vi "Configure Multi Eval Meas List Segment DMRS Type B.vi"(1 "Segment (1)":T3=1, 4 "Max Length (1)":i32=1, 5 "Additional Position (0)":i32, 6 "Config Type (1)":i32=1, 7 "Bandwidth Part (BWP0)":T1 items=["BWP0"], 8 "error in (no error)":errorcluster, 9 "Carrier Component (1)":T2=1, 10 "Instance (1)":T4=1, 11 "VISA resource name":refnum<visa-resource-name>) -> (0 "error out":errorcluster, 3 "VISA resource name out":refnum<visa-resource-name>)   [LabVIEW 2020, in "Rohde&Schwarz CMXP NR FR2 Measurement.lvlib"]
doc: "Configures the DM-RS for mapping type B. The settings apply to the <BWP> on carrier <cc> in segment <no>.\n\nAttribute:\nRSCMXPNRFR2M_ATTR_MULTI_EVAL_MEASUREMENT_LIST_SEGMENT_DMRS_TYPE_B\n\nRemote-control command:\nCONFigure:NRMMw:MEAS<i>:LIST:SEGMent<no>[:CC<cc>]:BWPart:PUSCh:DMTB"
uses:
  <instrlib>/Rohde&Schwarz CMXP NR FR2 Measurement/Rohde&Schwarz CMXP NR FR2 Measurement.lvlib
  <instrlib>/Rohde&Schwarz CMXP NR FR2 Measurement/Private/_Instance.ctl
  <instrlib>/Rohde&Schwarz CMXP NR FR2 Measurement/Private/_Segment.ctl
  <instrlib>/Rohde&Schwarz CMXP NR FR2 Measurement/Private/_Carrier Component.ctl
  <instrlib>/Rohde&Schwarz CMXP NR FR2 Measurement/Private/_Bandwidth Part.ctl
  <instrlib>/Rohde&Schwarz CMXP NR FR2 Measurement/Private/rsidr_core.llb/rsidr_core.lvlib
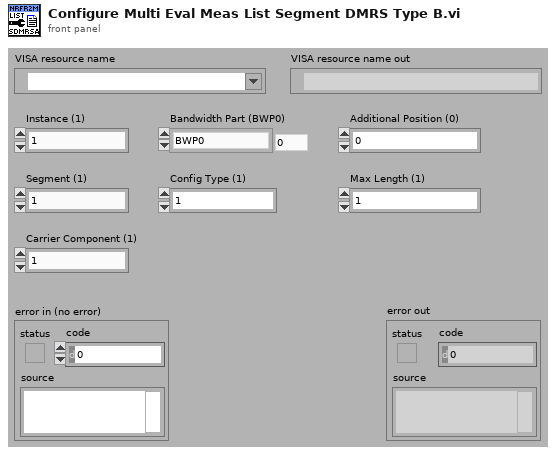
[diagram p1: front panel]
types:
  T1 = typedef "Rohde&Schwarz CMXP NR FR2 Measurement.lvlib/_Bandwidth Part.ctl" = i32
  T2 = typedef "Rohde&Schwarz CMXP NR FR2 Measurement.lvlib/_Carrier Component.ctl" = i32
  T3 = typedef "Rohde&Schwarz CMXP NR FR2 Measurement.lvlib/_Segment.ctl" = i32
  T4 = typedef "Rohde&Schwarz CMXP NR FR2 Measurement.lvlib/_Instance.ctl" = i32
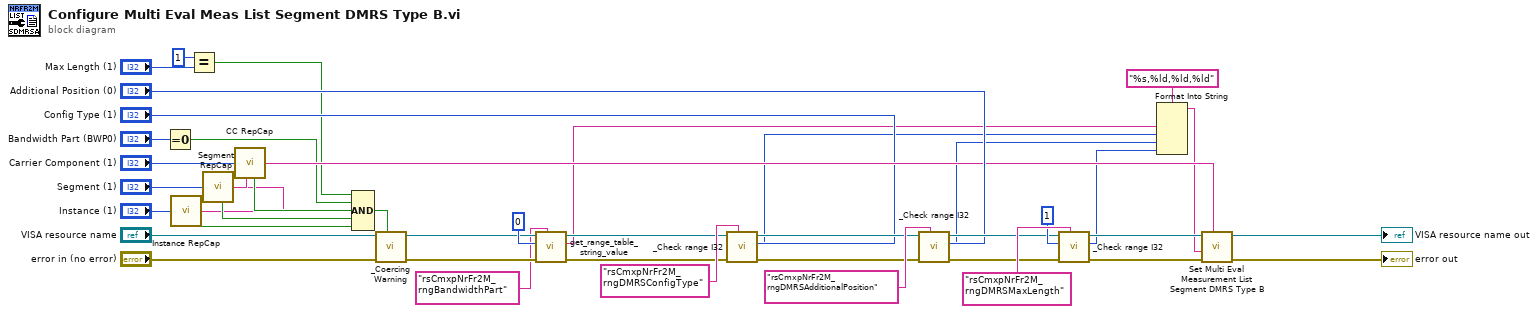
[diagram p0: block diagram]
diagram:
  n1 = Equal To 0?(x="Bandwidth Part (BWP0)") -> (x = 0?=w5:bool)
  n2 = call <instrlib>:"Instance RepCap.vi"("Instance In"="Instance (1)") -> ("In Range?"=w26:bool, "RepCap Identifier Out"=w2:string)  [unwired: 1 in]
  n3 = Equal?(x=1, y="Max Length (1)") -> (x = y?=w4:bool)
  n4 = call <instrlib>:"Segment RepCap.vi"("Segment In"="Segment (1)", "RepCap String In (\"\")"=w2) -> ("In Range?"=w25:bool, "RepCap Identifier Out"=w24:string)
  n5 = call <instrlib>:"CC RepCap.vi"("CC In"="Carrier Component (1)", "RepCap String In (\"\")"=w24) -> ("In Range?"=w23:bool, "RepCap Identifier Out"=w11:string)
  n6 = Compound Arithmetic op=AND(w4, w5, w23, w25, w26) -> (w29:bool)
  n7 = call <instrlib>:"_Coercing Warning.vi"("In Range?"=w29, "error in (no error)"="error in (no error)", "VISA resource name"="VISA resource name") -> ("error out"=w19:errorcluster, "VISA resource name out"=w18:refnum<visa-resource-name>)  [unwired: 7 in]
  n8 = call <instrlib>:"get_range_table_string_value.vi"("Range Table ID in"="rsCmxpNrFr2M_rngBandwidthPart", "error in"=w19, "I32 input"=0, "VISA resource name"=w18) -> ("error out"=w33:errorcluster, "String Value out"=w9:string, "VISA resource name out"=w32:refnum<visa-resource-name>)  [unwired: 5 in]
  n9 = call <instrlib>:"_Check range I32.vi"("Range Table Identifier"="rsCmxpNrFr2M_rngDMRSConfigType", "error in (no error)"=w33, "I32 Value In"="Config Type (1)", "VISA resource name"=w32) -> ("error out"=w40:errorcluster, "I32 Value Out"=w8:i32, "VISA resource name out"=w39:refnum<visa-resource-name>)  [unwired: 5 in]
  n10 = call <instrlib>:"_Check range I32.vi"("Range Table Identifier"="rsCmxpNrFr2M_rngDMRSAdditionalPosition", "error in (no error)"=w40, "I32 Value In"="Additional Position (0)", "VISA resource name"=w39) -> ("error out"=w36:errorcluster, "I32 Value Out"=w7:i32, "VISA resource name out"=w35:refnum<visa-resource-name>)  [unwired: 5 in]
  n11 = call <instrlib>:"_Check range I32.vi"("Range Table Identifier"="rsCmxpNrFr2M_rngDMRSMaxLength", "error in (no error)"=w36, "I32 Value In"=1, "VISA resource name"=w35) -> ("error out"=w14:errorcluster, "I32 Value Out"=w6:i32, "VISA resource name out"=w15:refnum<visa-resource-name>)  [unwired: 5 in]
  n12 = Format Into String(format string="%s,%ld,%ld,%ld", w9, w8, w7, w6) -> (resulting string=w1:string)  [unwired: 2 in, 1 out]
  n13 = call "Set Multi Eval Measurement List Segment DMRS Type B"("Repeated Capabilities"=w11, "error in (no error)"=w14, "Multi Eval Measurement List Segment DMRS Type B ()"=w1, "instrument handle"=w15) -> ("error out"=→"error out":errorcluster, "instrument handle out"=→"VISA resource name out":refnum<visa-resource-name>)  [unwired: 6 in]
